vi "Swp_Main.vi"() -> ()   [LabVIEW 2024]
panel:
  out "输出日志 log":string
  in  "响应端口额外频率位移":i8(ring) items=["-2次基波"=-2, "-1次基波"=-1, "无位移"=0, "+1次基波"=1, "+2次基波"=2, "对称-2次基波"=98, "对称-1次基波"=99, "对称"=100, "对称+1次基波"=101, "对称+2次基波"=102]
  in  "响应(2号)端口类型":u8(ring) items=["单相", "三相αβ系", "三相同步系", "三相正负序"]
  in  "测量模式":u8(ring)=1 items=["仅测量信号", "扫频"]
  in  "与DSP连接的串口":refnum<visa-resource-name>
  in  "同步相位来源":u8(ring) items=["1号A相", "2号A相"]
  in  "检验示波器":bool
  in  "错误常量":errorcluster
  in  "DSP同时注入频点数":u32=5 min=1 max=20
  out "csv中存储列分别为":string
  in  "触发方向":u16(ring)=2 items=["Rising"=2, "Falling"=3]
  in  "触发阈值 (V)":dbl min=-20.0 max=20.0
  in  "示波器量程":u16(ring)=10 items=["20 mV"=1, "50 mV"=2, "100 mV"=3, "200 mV"=4, "500 mV"=5, "1 V"=6, "2 V"=7, "5 V"=8, "10 V"=9, "20 V"=10]
  out "测试选项说明":string
  in  "基波频率 f_fun":u32=50 min=1 max=100000
  in  "注入(1号)端口类型":u8(ring) items=["单相", "三相αβ系", "三相同步系", "三相正负序"]
  in  "实际幅值 Amp":u8(ring)=1 items=["= Amp0", "= Amp0 / freq"]
  in  "默认幅值 Amp0":u8(ring)=2 items=["10.0", "5.0", "1.0", "0.5", "0.1", "0.05", "0.01"]
  in  "等待稳态时间":dbl=0.04 min=1e-06 max=1.0
  out "Pha":cluster{dbl[], dbl[]}[](graph)
  out "Mag":cluster{dbl[], dbl[]}[](graph)
  in  "stop":bool
  out "PICOerror":bool
  in  "开始扫频":bool
  in  "总电源":bool=TRUE
  out "可以正常测量":bool
  out "正在扫频":bool
  in  "幅值显示方式":u8(ring) items=["dB", "abs"]
  in  "测量周期数 n":u32=2 min=1 max=10
  in  "同步频率上限 f_tick_ref":u32=1 min=1 max=50
  out "单频点最大使用内存":u64 caption="单频点最大使用内存(kS)"
  out "扫频点预览":cluster{"freqs":i32[], "freqs":dbl[]}[](graph)
  out "实际有效频点数 N":i32
  in  "密集中心频率 f_dens":u32=50 min=1 max=1000000
  in  "密度常数 dens":dbl min=0.0 max=50.0
  out "扫频点报告":string
  in  "期望频点数 N0":u32=20 min=2
  in  "频率下限 f_min":u32=10 min=1 max=500000
  in  "频率上限 f_max":u32=5000 min=10 max=1000000
  # "版本：v1.1 允许异性端口的扫频。允许在DSP或PICO未连接时跳过通信或采样环节。"
  # "如果你后续要增加端口类型选项，请不要改动现存项对应的取值。"
  # "操作面板"
  # "频点生成设置"
  # "频点采样设置"
  # "响应测试模式设置"
  # "示波器设置"
  # "基础设置\n实际频点生成也与测试模式相关。"
  # "Hz"
  # "程序总开关"
  # "频率越低，耗时越长。精度越高。"
  # "Hz"
  # "Hz"
  # "kS"
  # "完成设置后，按下以扫频。\n期间锁定操作。"
  # "Hz"
  # "默认测量所有4通道。\n\n例如，在测量 2500 Hz 响应时，\n总时长可以是 1 s，也可以是 1e-3 s。\n\nf_tick_ref 表示采样总时长的下限。\n不建议设置高于低频次谐波。"
  # "密度设置（测试功能）\n设为 dens<1.0 以禁用"
  # "通信设置"
  # "V"
  # "Hz"
  # "强制退出扫频。它不会被锁"
  # "s"
  # "杂项输出显示"
  # "扫频结果显示"
  # "测试面板，仅供开发过程中使用。"
  # "存储至csv时总是abs."
  # "与DSP间通信方式：\n\n开启串口\n送出1字节FFFF，以提醒DSP，接下来要进入允许输出的模式\n等待回应1字节（内容不限），以确认已建立联系\n\n第k次扫频循环中：\n送出1字节FF00，以提醒DSP，接下来要输出一组频率\n第1频点A相频率输出（1字节，16位无符号整型）\n第1频点A相幅值输出（2字节，32位浮点数）\n第1频点A相相位输出（1字节，16位无符号整型，360角度制）\n第1频点B相频率\n第1频点B相幅值\n第1频点B相相位\n第1频点C相频率\n第1频点C相幅值\n第1频点C相相位\n第2频点……\n……\n第n频点……\n送出1字节FF00，以表示这一组频点已经发送完毕\n等待DSP回应1字节，确认DSP已收到指令\n等待一段时间，该时间可在主界面内设置\n\n送出1字节F000，以提醒DSP，接下来要结束了\n等待DSP回应1字节，确认DSP知道要关闭了\n关闭串口\n\n备注：如果已知DSP可接收的最大频点数，请设置在该界面内。\n通信中，多余的频点位会用全0补齐。"
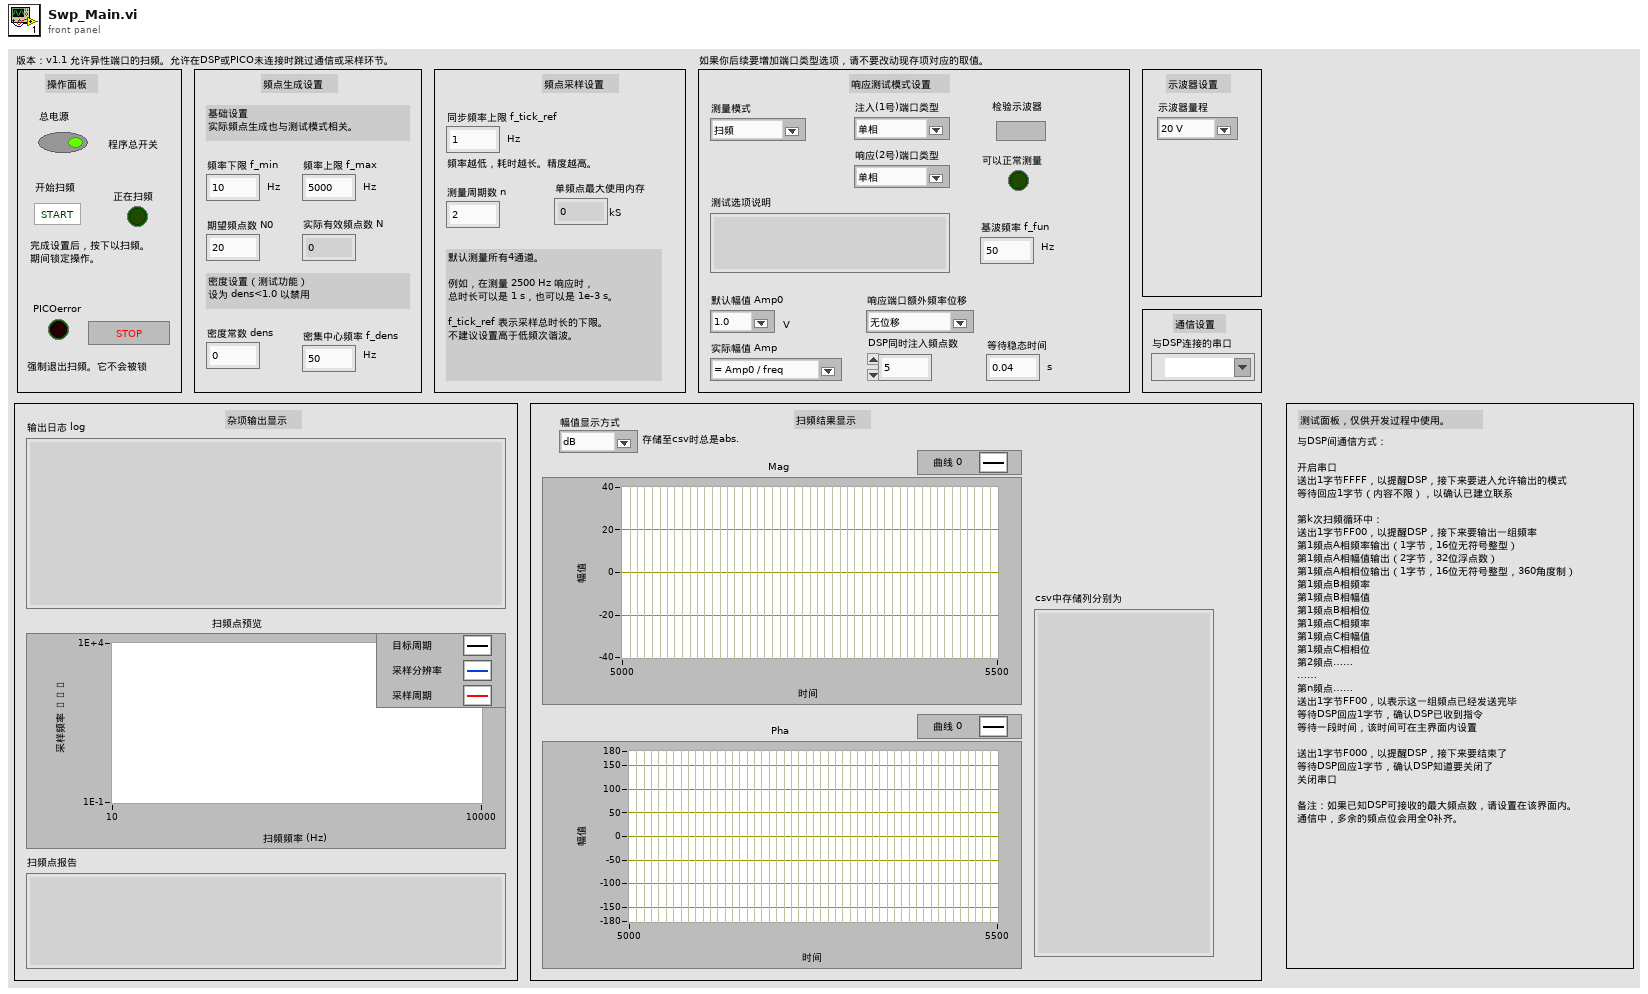
[diagram p1: front panel]
types:
  T1 = enum8{"Enabled", "Disabled", "Disabled and Grayed Out"}
  T2 = cluster{u32, u32, u32, dbl, u32, u8, u8, u8, u32, u32, u32, u32}
  T3 = enum16{"open", "replace", "create", "open or create", "replace or create", "replace or create with confirmation"}
  T4 = cluster{"Device Info":cluster{"Driver Version":string, "USB Version":string, "Hardware":string, "Variant":string, "Batch and Serial":string, "Cal Date":string, "Kernel Version":string, "Digital HW Version":string, "Analogue HW Version":string, "Firmware 1":string, "Firmware 2":string, "MSO":bool, "Number of Channels":i16}, "error out":errorcluster, "handle out":i16, "Enabled Array":i16[], "Max Adc value":i16}[]
  T5 = cluster{"Device Info":cluster{"Driver Version":string, "USB Version":string, "Hardware":string, "Variant":string, "Batch and Serial":string, "Cal Date":string, "Kernel Version":string, "Digital HW Version":string, "Analogue HW Version":string, "Firmware 1":string, "Firmware 2":string, "MSO":bool, "Number of Channels":i16}, "error out":errorcluster, "handle out":i16, "Enabled Array":i16[], "Max Adc value":i16}
  T6 = cluster{"Driver Version":string, "USB Version":string, "Hardware":string, "Variant":string, "Batch and Serial":string, "Cal Date":string, "Kernel Version":string, "Digital HW Version":string, "Analogue HW Version":string, "Firmware 1":string, "Firmware 2":string, "MSO":bool, "Number of Channels":i16}
  T7 = cluster{"Device Info":cluster{"Driver Version":string, "USB Version":string, "Hardware":string, "Variant":string, "Batch and Serial":string, "Cal Date":string, "Kernel Version":string, "Digital HW Version":string, "Analogue HW Version":string, "Firmware 1":string, "Firmware 2":string, "MSO":bool, "Number of Channels":i16}, "Enabled Array":i16[], "handle out":i16, "error out":errorcluster}
  T8 = cluster{"Channel A Buffer":i16[], "Channel B Buffer":i16[], "Channel C Buffer":i16[], "Channel D Buffer":i16[], "Channel E Buffer":i16[], "Channel F Buffer":i16[], "Channel G Buffer":i16[], "Channel H Buffer":i16[], "Port 0 Buffer":i16[], "Port 1 Buffer":i16[]}[]
  T9 = typedef "PicoBuffers.ctl" = cluster{"Max Buffer Pointers":u64[][][], "Min Buffer Pointers":u64[][][], "StreamingDataInfo":cluster{"Channel":u32, "Down-Sample Mode":u32, "PICO_DATA_TYPE":enum32{"PICO_INT8_T", "PICO_INT16_T", "PICO_INT32_T", "PICO_UINT32_T", "PICO_INT64_T", ""}, "Samples":i32, "bufferIndex":u64, "startIndex":i32, "overflow":i16}[][]}
  T10 = cluster{"Data Pointers":T9, "error out":errorcluster, "handle out":i16}
  T11 = cluster{"Data":dbl[], "Data":dbl[], "Data":dbl[], "Data":dbl[], "Data":dbl[], "Data":dbl[]}
  T12 = cluster{"Data Pointers":T9, "Enabled Array":i16[], "error out":errorcluster, "handle out":i16}
  T13 = cluster{"Data Pointers":T9, "Enabled Array":i16[], "error out":errorcluster, "handle out":i16}[]
  T14 = cluster{"Value":u32, "Value":u32, "Value":u32, "Value":dbl, "Value":u32, "Value":u8, "Value":u8, "Value":u8, "Value":u32, "Value":u32, "Value":u32, "Value":u32}
  T15 = cluster{bool, bool, bool, bool, bool, bool, bool, bool, bool, bool, bool, bool}
  T16 = cluster{"freqs, measu, measu comp":i32[], dbl[]}[]
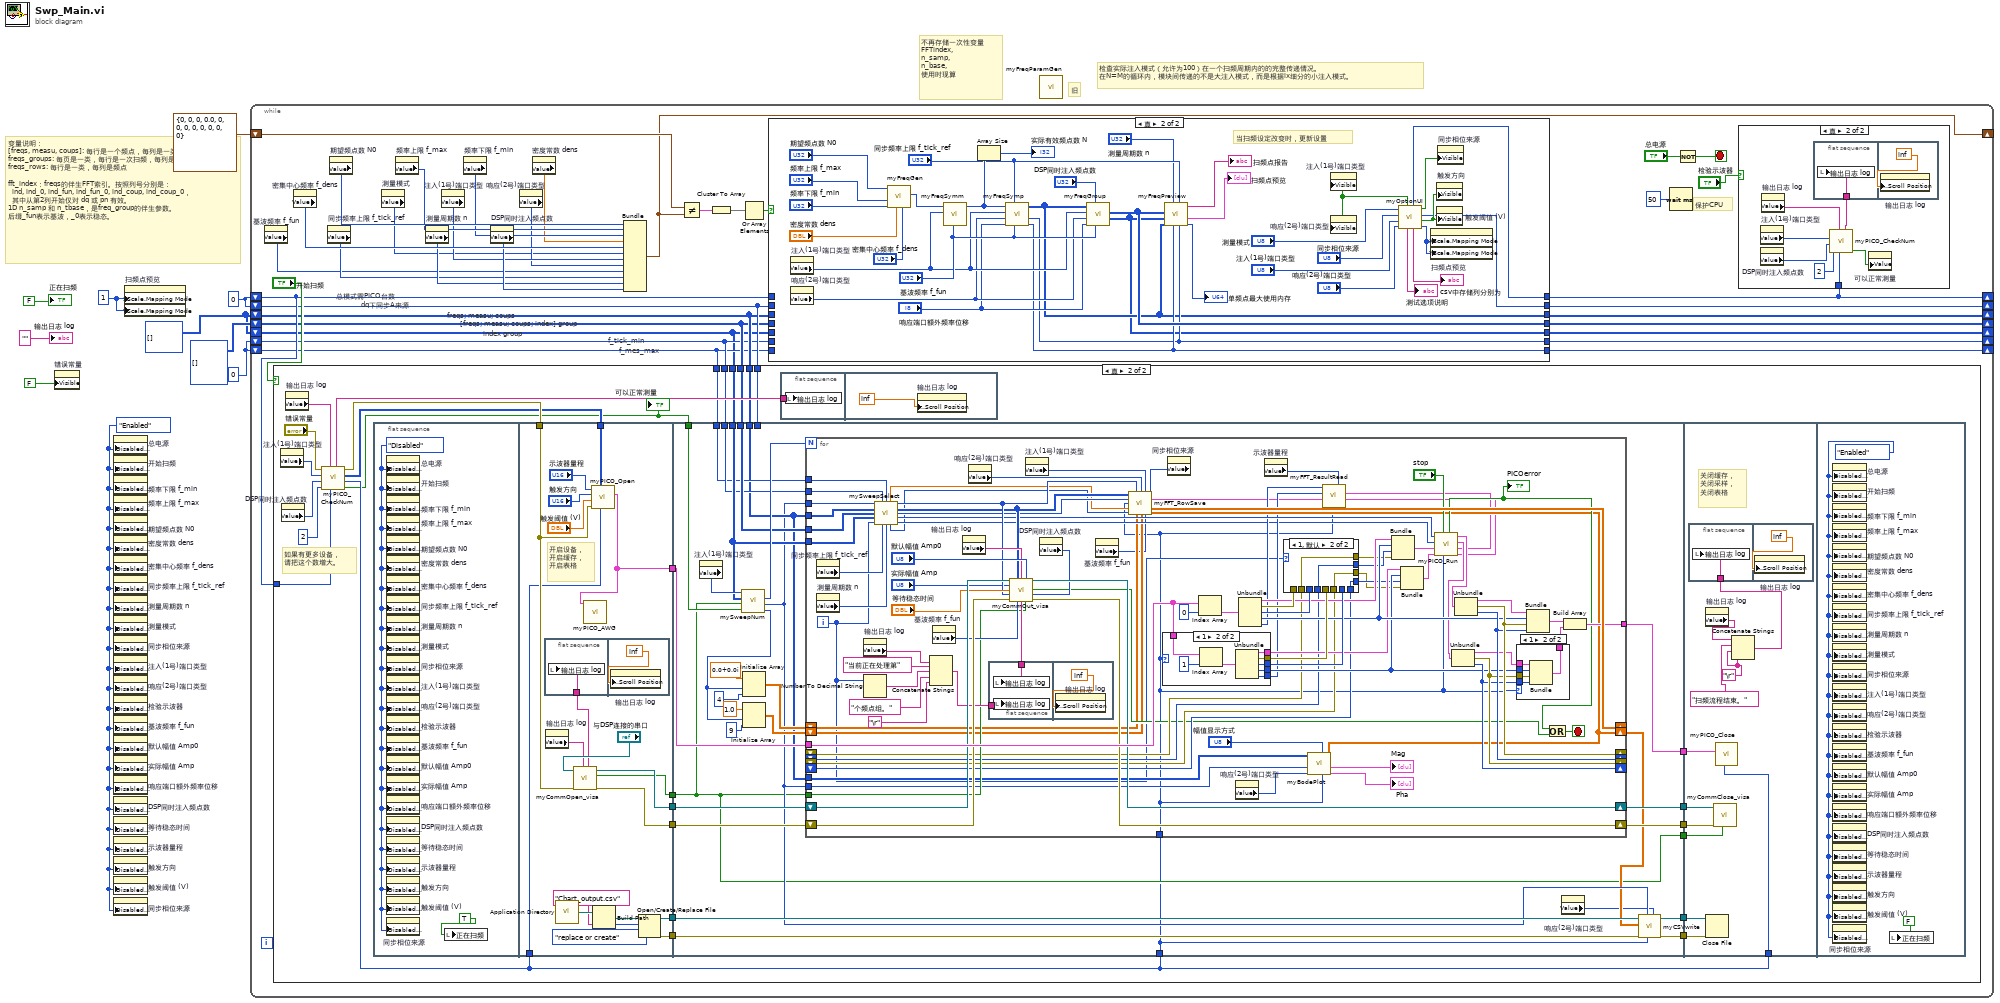
[diagram p0: block diagram]
diagram:
  w3 = u32 0
  w5 = u8 1 ("X标尺.映射模式")
  w6 = T1."Enabled" ("禁用")
  w8 = u8 0
  w1 = i32[][] []
  # "不再存储一次性变量\nFFTindex, \nn_samp, \nn_base, \n使用时现算"
  # "检查实际注入模式（允许为100）在一个扫频周期内的的完整传递情况。\n在N=M的循环内，模块间传递的不是大注入模式，而是根据ix细分的小注入模式。"
  # "旧"
  # "变量说明：\n[freqs, measu, coups]: 每行是一个频点，每列是一类\nfreqs_groups: 每页是一类，每行是一次扫频，每列是频点\nfreqs_rows: 每行是一类，每列是频点\n\nfft_index：freqs的伴生FFT索引。按照列号分别是：\n  ind, ind_0, ind_fun, ind_fun_0, ind_coup, ind_coup_0，\n  其中从第2列开始仅对 dq 或 pn 有效。\n1D n_samp 和 n_tbase，是freq_group的伴生参数。\n后缀_fun表示基波，_0表示稳态。"
  n1 = property on="错误常量" class="Clust (严格)"("Visible"=FALSE ("可见")) -> ()  [unwired: 2 in, 2 out]
  n2 = property on="总电源" class="Bool"("DisabledEnum"=w6) -> ()  [unwired: 2 in, 2 out]
  n3 = property on="开始扫频" class="Bool"("DisabledEnum"=w6) -> ()  [unwired: 2 in, 2 out]
  n4 = property on="频率下限 f_min" class="DigNum (严格)"("DisabledEnum"=w6) -> ()  [unwired: 2 in, 2 out]
  n5 = property on="频率上限 f_max" class="DigNum (严格)"("DisabledEnum"=w6) -> ()  [unwired: 2 in, 2 out]
  n6 = property on="期望频点数 N0" class="DigNum (严格)"("DisabledEnum"=w6) -> ()  [unwired: 2 in, 2 out]
  n7 = property on="密度常数 dens" class="DigNum (严格)"("DisabledEnum"=w6) -> ()  [unwired: 2 in, 2 out]
  n8 = property on="密集中心频率 f_dens" class="DigNum (严格)"("DisabledEnum"=w6) -> ()  [unwired: 2 in, 2 out]
  n9 = property on="同步频率上限 f_tick_ref" class="DigNum (严格)"("DisabledEnum"=w6) -> ()  [unwired: 2 in, 2 out]
  n10 = property on="测量周期数 n" class="DigNum (严格)"("DisabledEnum"=w6) -> ()  [unwired: 2 in, 2 out]
  n11 = property on="测量模式" class="Ring (严格)"("DisabledEnum"=w6) -> ()  [unwired: 2 in, 2 out]
  n12 = property on="同步相位来源" class="Ring (严格)"("DisabledEnum"=w6) -> ()  [unwired: 2 in, 2 out]
  n13 = property on="注入(1号)端口类型" class="Ring (严格)"("DisabledEnum"=w6) -> ()  [unwired: 2 in, 2 out]
  n14 = property on="响应(2号)端口类型" class="Ring (严格)"("DisabledEnum"=w6) -> ()  [unwired: 2 in, 2 out]
  n15 = property on="检验示波器" class="Bool"("DisabledEnum"=w6) -> ()  [unwired: 2 in, 2 out]
  n16 = property on="基波频率 f_fun" class="DigNum (严格)"("DisabledEnum"=w6) -> ()  [unwired: 2 in, 2 out]
  n17 = property on="默认幅值 Amp0" class="Ring (严格)"("DisabledEnum"=w6) -> ()  [unwired: 2 in, 2 out]
  n18 = property on="实际幅值 Amp" class="Ring (严格)"("DisabledEnum"=w6) -> ()  [unwired: 2 in, 2 out]
  n19 = property on="响应端口额外频率位移" class="Ring (严格)"("DisabledEnum"=w6) -> ()  [unwired: 2 in, 2 out]
  n20 = property on="DSP同时注入频点数" class="DigNum (严格)"("DisabledEnum"=w6) -> ()  [unwired: 2 in, 2 out]
  n21 = property on="等待稳态时间" class="DigNum (严格)"("DisabledEnum"=w6) -> ()  [unwired: 2 in, 2 out]
  n22 = property on="示波器量程" class="Ring (严格)"("DisabledEnum"=w6) -> ()  [unwired: 2 in, 2 out]
  n23 = property on="触发方向" class="Ring (严格)"("DisabledEnum"=w6) -> ()  [unwired: 2 in, 2 out]
  n24 = property on="触发阈值 (V)" class="DigNum (严格)"("DisabledEnum"=w6) -> ()  [unwired: 2 in, 2 out]
  n25 = property on="同步相位来源" class="Ring (严格)"("DisabledEnum"=w6) -> ()  [unwired: 2 in, 2 out]
  n26 = property on="扫频点预览" class="XYGraph (严格)"("XScale.Mapping Mode"=w5, "YScale.Mapping Mode"=w5) -> ()  [unwired: 2 in, 2 out]
  n27 = while {
    shift-right: [w37] -> _
    shift-left: T2 {0, 0, 0, 0.0, 0, 0, 0, 0, 0, 0, 0, 0} -> [w38]
    shift-right: [w32] -> _
    shift-left: w1 -> [w17]
    shift-right: [w24] -> _
    shift-left: w8 -> [w20]
    shift-right: [w23] -> _
    shift-left: w8 -> [w18]
    shift-right: [w22] -> _
    shift-left: w3 -> [w15]
    shift-right: [w21] -> _
    shift-left: w3 -> [w14]
    shift-right: [w19] -> _
    shift-left: i32[][][] [] -> [w16]
    shift-right: [w13] -> _
    shift-left: w1 -> [w12]
    stop <- w45 stop-if-true
    # "index group"
    # "f_mes_max"
    # "f_tick_min"
    # "[freqs; measu; coups; index] group"
    # "freqs; measu; coups"
    # "总模式需PICO台数"
    # "dq下同步A来源"
    # "保护CPU"
    n28 = property on="基波频率 f_fun" class="DigNum (严格)"() -> ("Value"=w28:u32)  [unwired: 2 in, 2 out]
    n29 = case shown="真" "开始扫频" {
      tunnel: w20 -> [_ w118]
      tunnel: w18 -> [_ w98]
      tunnel: w17 -> [_ w99]
      tunnel: w16 -> [_ w100]
      tunnel: w15 -> [_ w101]
      tunnel: w14 -> [_ w102]
      tunnel: w12 -> [_ w103]
      frame False {
      }
      frame True {
        # "如果有更多设备，\n请把这个数增大。"
        n30 = property on="注入(1号)端口类型" class="Ring (严格)"() -> ("Value"=w122:u8)  [unwired: 2 in, 2 out]
        n31 = property on="DSP同时注入频点数" class="DigNum (严格)"() -> ("Value"=w121:u32)  [unwired: 2 in, 2 out]
        n32 = property on="输出日志 log" class="Str"() -> ("Value"=w120:string)  [unwired: 2 in, 2 out]
        n33 = call "myPICO_CheckNum.vi"("需要的示波器台数"=w118, "当前log"=w120, "最大检测设备数"=i16 2, "最大同时扫频数"=w121, "注入(1号)端口类型"=w122, "错误常量"="错误常量") -> ("可以正常测量"=w104:bool, "实际驱动设备数"=w105:u16, "序列号组 2"=w123:i8[][], "错误输出"=w124:errorcluster, "更新log"=w119:string)  [unwired: 1 in]
        "可以正常测量" <- w104
        n34 = flat-sequence {
          tunnel: w123 -> [w147]
          tunnel: w124 -> [w137]
          tunnel: [w133] -> w117
          tunnel: [w139] -> w116
          tunnel: [w138] -> w115
          tunnel: [w135] -> w114
          tunnel: [w134] -> w113
          tunnel: w105 -> [w130]
          tunnel: [w129] -> w112
          tunnel: w117 -> [w174]
          tunnel: w105 -> [w150]
          tunnel: [w173] -> w111
          tunnel: w116 -> [w165]
          tunnel: w115 -> [w172]
          tunnel: [w166] -> w110
          tunnel: [w171] -> w109
          tunnel: w114 -> [w170]
          tunnel: w113 -> [w169]
          tunnel: [w168] -> w108
          tunnel: [w167] -> w107
          tunnel: w112 -> [w152]
          tunnel: [w152] -> w106
          tunnel: w104 -> [w162]
          tunnel: w103 -> [w160]
          tunnel: w102 -> [w158]
          tunnel: w101 -> [w159]
          tunnel: w100 -> [w161]
          tunnel: w99 -> [w157]
          tunnel: w98 -> [_]
          tunnel: w105 -> [w295]
          tunnel: w111 -> [w305]
          tunnel: w110 -> [w304]
          tunnel: w109 -> [w303]
          tunnel: w108 -> [w302]
          tunnel: w107 -> [w301]
          tunnel: w106 -> [w296]
          frame #0 {
            w128 = T1."Disabled" ("禁用")
            n35 = property on="总电源" class="Bool"("DisabledEnum"=w128) -> ()  [unwired: 2 in, 2 out]
            n36 = property on="开始扫频" class="Bool"("DisabledEnum"=w128) -> ()  [unwired: 2 in, 2 out]
            n37 = property on="频率下限 f_min" class="DigNum (严格)"("DisabledEnum"=w128) -> ()  [unwired: 2 in, 2 out]
            n38 = property on="频率上限 f_max" class="DigNum (严格)"("DisabledEnum"=w128) -> ()  [unwired: 2 in, 2 out]
            n39 = property on="期望频点数 N0" class="DigNum (严格)"("DisabledEnum"=w128) -> ()  [unwired: 2 in, 2 out]
            n40 = property on="密度常数 dens" class="DigNum (严格)"("DisabledEnum"=w128) -> ()  [unwired: 2 in, 2 out]
            n41 = property on="密集中心频率 f_dens" class="DigNum (严格)"("DisabledEnum"=w128) -> ()  [unwired: 2 in, 2 out]
            n42 = property on="同步频率上限 f_tick_ref" class="DigNum (严格)"("DisabledEnum"=w128) -> ()  [unwired: 2 in, 2 out]
            n43 = property on="测量周期数 n" class="DigNum (严格)"("DisabledEnum"=w128) -> ()  [unwired: 2 in, 2 out]
            n44 = property on="测量模式" class="Ring (严格)"("DisabledEnum"=w128) -> ()  [unwired: 2 in, 2 out]
            n45 = property on="同步相位来源" class="Ring (严格)"("DisabledEnum"=w128) -> ()  [unwired: 2 in, 2 out]
            n46 = property on="注入(1号)端口类型" class="Ring (严格)"("DisabledEnum"=w128) -> ()  [unwired: 2 in, 2 out]
            n47 = property on="响应(2号)端口类型" class="Ring (严格)"("DisabledEnum"=w128) -> ()  [unwired: 2 in, 2 out]
            n48 = property on="检验示波器" class="Bool"("DisabledEnum"=w128) -> ()  [unwired: 2 in, 2 out]
            n49 = property on="基波频率 f_fun" class="DigNum (严格)"("DisabledEnum"=w128) -> ()  [unwired: 2 in, 2 out]
            n50 = property on="默认幅值 Amp0" class="Ring (严格)"("DisabledEnum"=w128) -> ()  [unwired: 2 in, 2 out]
            n51 = property on="实际幅值 Amp" class="Ring (严格)"("DisabledEnum"=w128) -> ()  [unwired: 2 in, 2 out]
            n52 = property on="响应端口额外频率位移" class="Ring (严格)"("DisabledEnum"=w128) -> ()  [unwired: 2 in, 2 out]
            n53 = property on="DSP同时注入频点数" class="DigNum (严格)"("DisabledEnum"=w128) -> ()  [unwired: 2 in, 2 out]
            n54 = property on="等待稳态时间" class="DigNum (严格)"("DisabledEnum"=w128) -> ()  [unwired: 2 in, 2 out]
            n55 = property on="示波器量程" class="Ring (严格)"("DisabledEnum"=w128) -> ()  [unwired: 2 in, 2 out]
            n56 = property on="触发方向" class="Ring (严格)"("DisabledEnum"=w128) -> ()  [unwired: 2 in, 2 out]
            n57 = property on="触发阈值 (V)" class="DigNum (严格)"("DisabledEnum"=w128) -> ()  [unwired: 2 in, 2 out]
            n58 = property on="同步相位来源" class="Ring (严格)"("DisabledEnum"=w128) -> ()  [unwired: 2 in, 2 out]
            n59 = local write "正在扫频"(TRUE) -> ()
          }
          frame #1 {
            # "开启设备，\n开启缓存，\n开启表格"
            n60 = flat-sequence {
              tunnel: w131 -> [w148]
              frame #0 {
                n61 = local write "输出日志 log"(w148) -> ()
              }
              frame #1 {
                n62 = property on="输出日志 log" class="Str"("Text.Scroll Position"=inf) -> ()  [unwired: 2 in, 2 out]
              }
            }
            n63 = property on="输出日志 log" class="Str"() -> ("Value"=w132:string)  [unwired: 2 in, 2 out]
            n64 = call <vilib>:"Application Directory.vi"() -> ("Application Directory"=w142:path)
            n65 = call "myCommOpen_visa.vi"("log输入"=w132, "错误输入（无错误）"=w137, "与DSP连接的串口"="与DSP连接的串口") -> ("错误输出"=w134:errorcluster, "是否有可用DSP"=w129:bool, "VISA resource name out"=w135:refnum<visa-resource-name>, "log输出"=w131:string)  [unwired: 5 in]
            n66 = call "myPICO_Open.vi"("需要台数"=w130, "serials"=w147, "错误输入（无错误）"=w137, "触发阈值 (V)"="触发阈值 (V)", "触发方向"="触发方向", "示波器量程"="示波器量程") -> ("数组"=w133:T4)  [unwired: 5 in]
            n67 = call "myPICO_AWG.vi"("数组"=w133) -> ()  [unwired: 11 in]
            n68 = Build Path(base path=w142, name or relative path="Chart_output.csv" ("name (excel)")) -> (appended path=w141:path)
            n69 = Open/Create/Replace File(file path (use dialog)=w141, operation (0:open)=T3."replace or create" ("操作(0:open)")) -> (refnum out=w139:refnum<file>, error out=w138:errorcluster)  [unwired: 4 in, 1 out]
          }
          frame #2 {
            n70 = property on="注入(1号)端口类型" class="Ring (严格)"() -> ("Value"=w163:u8)  [unwired: 2 in, 2 out]
            n71 = call "mySweepNum.vi"("可以正常测量"=w162, "是否有可用DSP"=w152, "index group"=w160, "注入(1号)端口类型"=w163) -> ("频点数"=w156:i32, "实际使用的注入模式"=w154:u8, "M"=w164:i32)  [unwired: 5 in]
            n72 = Initialize Array(cdb 0.0+0.0i, w156, 4 ("维数大小")) -> (w176:cdb[][])
            n73 = Initialize Array(1.0 ("元素"), w156, 9 ("维数大小")) -> (w175:dbl[][])
            n74 = for {
              N: w164 -> [_]
              shift-right: [w270] -> _
              shift-left: w176 -> [w186]
              shift-right: [w202] -> w153
              shift-left: w175 -> [w187]
              shift-right: [w269] -> _
              shift-left: _ -> [w207]
              shift-right: [w268] -> _
              shift-left: _ -> [w206]
              shift-right: [w267] -> _
              shift-left: _ -> [w205]
              shift-right: [w266] -> _
              shift-left: _ -> [w204]
              tunnel: w150 -> [w180]
              tunnel: w174 -> [w264]
              tunnel: [w265] -> w173
              shift-right: [w256] -> w167
              shift-left: w170 -> [w261]
              shift-right: [w257] -> w168
              shift-left: w169 -> [w260]
              tunnel: w152 -> [w213]
              tunnel: w154 -> [w221]
              tunnel: w157 -> [w220]
              tunnel: w161 -> [w219]
              tunnel: w160 -> [w218]
              tunnel: w159 -> [w215]
              tunnel: w158 -> [w214]
              tunnel: w154 -> [w199]
              tunnel: w157 -> [w201]
              i -> [w181]
              stop <- w258 stop-if-true
              n75 = property on="同步频率上限 f_tick_ref" class="DigNum (严格)"() -> ("Value"=w217:u32)  [unwired: 2 in, 2 out]
              n76 = property on="测量周期数 n" class="DigNum (严格)"() -> ("Value"=w216:u32)  [unwired: 2 in, 2 out]
              n77 = property on="输出日志 log" class="Str"() -> ("Value"=w247:string)  [unwired: 2 in, 2 out]
              n78 = Number To Decimal String(number=w181) -> (decimal integer string=w255:string)  [unwired: 1 in]
              n79 = call "mySweepSelect.vi"("实际使用的注入模式"=w221, "f_tick_min"=w215, "f_mes_max"=w214, "freqs, measu. coups"=w220, "freqs groups"=w219, "index group"=w218, "ix"=w181, "同步频率上限 f_tick_ref"=w217, "测量周期数 n"=w216) -> ("f_tick"=w185:dbl, "注入小模式"=w212:u8, "freq rows"=w211:i32[][], "index row"=w210:i32[], "sample"=w208:u64, "f_mes"=w184:i32, "timebase"=w189:u32)
              n80 = Concatenate Strings(w247, "当前正在处理第", w255, "个频点组。", "\r") -> (w246:string)
              n81 = property on="基波频率 f_fun" class="DigNum (严格)"() -> ("Value"=w249:u32)  [unwired: 2 in, 2 out]
              n82 = property on="输出日志 log" class="Str"() -> ("Value"=w244:string)  [unwired: 2 in, 2 out]
              n83 = property on="响应(2号)端口类型" class="Ring (严格)"() -> ("Value"=w190:u8)  [unwired: 2 in, 2 out]
              n84 = flat-sequence {
                tunnel: w246 -> [w293]
                tunnel: w245 -> [w292]
                frame #0 {
                  n85 = local write "输出日志 log"(w292) -> ()
                  n86 = local write "输出日志 log"(w293) -> ()
                }
                frame #1 {
                  n87 = property on="输出日志 log" class="Str"("Text.Scroll Position"=inf) -> ()  [unwired: 2 in, 2 out]
                }
              }
              n88 = property on="注入(1号)端口类型" class="Ring (严格)"() -> ("Value"=w183:u8)  [unwired: 2 in, 2 out]
              n89 = property on="DSP同时注入频点数" class="DigNum (严格)"() -> ("Value"=w248:u32)  [unwired: 2 in, 2 out]
              n90 = call "myCommOut_visa.vi"("VISA资源名称"=w261, "freqs rows"=w211, "log输入"=w244, "默认幅值 Amp0"="默认幅值 Amp0", "实际幅值 Amp"="实际幅值 Amp", "t_wait"="等待稳态时间", "扰动注入模式"=w212, "最大同时扫频数"=w248, "错误输入（无错误）"=w260, "基波频率"=w249, "存在DSP"=w213) -> ("VISA资源名称 2"=w256:refnum<visa-resource-name>, "error out"=w203:bool, "log输出"=w245:string, "错误输出"=w257:errorcluster)  [unwired: 1 in]
              n91 = property on="基波频率 f_fun" class="DigNum (严格)"() -> ("Value"=w182:u32)  [unwired: 2 in, 2 out]
              n92 = case shown="1" w180 {
                tunnel: w264 -> [_ w291]
                tunnel: [_ w290] -> w231
                tunnel: [_ w289] -> w238
                tunnel: [_ w288] -> w236
                tunnel: [_ w287] -> w192
                tunnel: [_ w284] -> w230
                frame 0, Default {
                }
                frame 1 {
                  n93 = Index Array(array=w291, index=1 ("索引")) -> (element=w285:T5)
                  n94 = Unbundle(w285) -> ("Device Info"=w290:T6, "error out"=w289:errorcluster, "handle out"=w288:i16, "Enabled Array"=w284:i16[], "Max Adc value"=w287:i16)
                }
              }
              n95 = property on="同步相位来源" class="Ring (严格)"() -> ("Value"=w209:u8)  [unwired: 2 in, 2 out]
              n96 = Index Array(array=w264, index=0 ("索引")) -> (element=w242:T5)
              n97 = property on="响应(2号)端口类型" class="Ring (严格)"() -> ("Value"=w198:u8)  [unwired: 2 in, 2 out]
              n98 = Unbundle(w242) -> ("Device Info"=w235:T6, "error out"=w239:errorcluster, "handle out"=w237:i16, "Enabled Array"=w234:i16[], "Max Adc value"=w193:i16)
              n99 = property on="示波器量程" class="Ring (严格)"() -> ("Value"=w191:u16)  [unwired: 2 in, 2 out]
              n100 = case shown="1, 默认" w181 {
                tunnel: w239 -> [w274 _]
                tunnel: w207 -> [_ w278]
                tunnel: w237 -> [w273 _]
                tunnel: w206 -> [_ w277]
                tunnel: w238 -> [w272 _]
                tunnel: w205 -> [_ w276]
                tunnel: w236 -> [w271 _]
                tunnel: w204 -> [_ w275]
                tunnel: [w274 w278] -> w232
                tunnel: [w273 w277] -> w233
                tunnel: [w272 w276] -> w228
                tunnel: [w271 w275] -> w229
                frame 0 {
                }
                frame 1, Default {
                }
              }
              n101 = Bundle("Device Info"=w235, "Enabled Array"=w234, "handle out"=w233, "error out"=w232) -> (w227:T7)  [unwired: 1 in]
              n102 = Bundle("Device Info"=w231, "Enabled Array"=w230, "handle out"=w229, "error out"=w228) -> (w226:T7)  [unwired: 1 in]
              n103 = call "myPICO_Run.vi"("实际驱动台数"=w180, "stop"="stop", "簇 3"=w226, "簇 4"=w227, "n_tbase"=w189, "n_samp"=w208) -> ("MultiBuffers (Max or non-aggregated) 2"=w194:T8, "MultiBuffers (Max or non-aggregated)"=w195:T8, "簇 2"=w197:T10, "簇"=w225:T10, "布尔输出"=w259:bool)  [unwired: 1 in]
              "PICOerror" <- w259
              n104 = call "myFFT_ResultRead.vi"("MultiBuffers 2"=w194, "MultiBuffers 1"=w195, "示波器量程"=w191, "可用示波器数"=w180, "Max Adc value 2"=w192, "Max Adc value"=w193) -> ("输出簇"=w188:T11)  [unwired: 5 in]
              n105 = call "myFFT_RowSave.vi"("freqs rows"=w211, "小注入模式"=w212, "响应模式"=w190, "注入(1号)端口类型"=w183, "dq同步来源"=w209, "index row"=w210, "采样结果簇"=w188, "可用pico数(仅用于模式100)"=w180, "f_tick"=w185, "f_mes"=w184, "稳态工作点输入"=w186, "写表结果输入"=w187, "基波频率 f_fun"=w182) -> ("稳态工作点输出"=w270:cdb[][], "写表结果输出"=w202:dbl[][])  [unwired: 1 in]
              n106 = call "myBodePlot.vi"("swp_data"=w202, "可用pico数"=w180, "幅值单位"="幅值显示方式", "响应选项"=w198, "注入选项"=w199, "freqs, meas, coups"=w201) -> ("Pha"=→"Pha":cluster{dbl[], dbl[]}[], "Mag"=→"Mag":cluster{dbl[], dbl[]}[])  [unwired: 4 in]
              n107 = Unbundle(w197) -> ("Data Pointers"=w224:T9, "error out"=w267:errorcluster, "handle out"=w266:i16)
              n108 = Unbundle(w225) -> ("Data Pointers"=w223:T9, "error out"=w269:errorcluster, "handle out"=w268:i16)
              n109 = case shown="1" w180 {
                tunnel: [_ w283] -> w241
                tunnel: w224 -> [_ w282]
                tunnel: w230 -> [_ w281]
                tunnel: w267 -> [_ w280]
                tunnel: w266 -> [_ w279]
                frame 0, Default {
                }
                frame 1 {
                  n110 = Bundle("Data Pointers"=w282, "Enabled Array"=w281, "error out"=w280, "handle out"=w279) -> (w283:T12)  [unwired: 1 in]
                }
              }
              n111 = Bundle("Data Pointers"=w223, "Enabled Array"=w234, "error out"=w269, "handle out"=w268) -> (w240:T12)  [unwired: 1 in]
              n112 = Or(x=w259, y=w203) -> (x .or. y?=w258:bool)
              n113 = Build Array(w240, w241) -> (w265:T13)
            }
            n114 = property on="响应(2号)端口类型" class="Ring (严格)"() -> ("Value"=w151:u8)  [unwired: 2 in, 2 out]
            n115 = call "myCSVwrite.vi"("响应选项"=w151, "可用PICO数"=w150, "注入选项"=w154, "错误输入（无错误）"=w172, "写表结果输入"=w153, "字节流文件输入"=w165) -> ("错误输出"=w171:errorcluster, "字节流文件输出"=w166:refnum<file>)  [unwired: 4 in]
          }
          frame #3 {
            w299 = "\r"
            # "关闭缓存，\n关闭采样，\n关闭表格"
            n116 = flat-sequence {
              tunnel: w297 -> [w306]
              frame #0 {
                n117 = local write "输出日志 log"(w306) -> ()
              }
              frame #1 {
                n118 = property on="输出日志 log" class="Str"("Text.Scroll Position"=inf) -> ()  [unwired: 2 in, 2 out]
              }
            }
            n119 = property on="输出日志 log" class="Str"() -> ("Value"=w298:string)  [unwired: 2 in, 2 out]
            n120 = Close File(refnum=w304, error in=w303) -> ()  [unwired: 2 out]
            n121 = call "myCommClose_visa.vi"("是否存在DSP"=w296, "错误输入（无错误）"=w302, "VISA资源名称"=w301) -> ()  [unwired: 8 in, 1 out]
            n122 = call "myPICO_Close.vi"("数值"=w295, "数组"=w305) -> ()  [unwired: 10 in]
            n123 = Concatenate Strings(w298, "扫频流程结束。", w299, w299) -> (w297:string)
          }
          frame #4 {
            w309 = T1."Enabled" ("禁用")
            n124 = property on="总电源" class="Bool"("DisabledEnum"=w309) -> ()  [unwired: 2 in, 2 out]
            n125 = property on="开始扫频" class="Bool"("DisabledEnum"=w309) -> ()  [unwired: 2 in, 2 out]
            n126 = property on="频率下限 f_min" class="DigNum (严格)"("DisabledEnum"=w309) -> ()  [unwired: 2 in, 2 out]
            n127 = property on="频率上限 f_max" class="DigNum (严格)"("DisabledEnum"=w309) -> ()  [unwired: 2 in, 2 out]
            n128 = property on="期望频点数 N0" class="DigNum (严格)"("DisabledEnum"=w309) -> ()  [unwired: 2 in, 2 out]
            n129 = property on="密度常数 dens" class="DigNum (严格)"("DisabledEnum"=w309) -> ()  [unwired: 2 in, 2 out]
            n130 = property on="密集中心频率 f_dens" class="DigNum (严格)"("DisabledEnum"=w309) -> ()  [unwired: 2 in, 2 out]
            n131 = property on="同步频率上限 f_tick_ref" class="DigNum (严格)"("DisabledEnum"=w309) -> ()  [unwired: 2 in, 2 out]
            n132 = property on="测量周期数 n" class="DigNum (严格)"("DisabledEnum"=w309) -> ()  [unwired: 2 in, 2 out]
            n133 = property on="测量模式" class="Ring (严格)"("DisabledEnum"=w309) -> ()  [unwired: 2 in, 2 out]
            n134 = property on="同步相位来源" class="Ring (严格)"("DisabledEnum"=w309) -> ()  [unwired: 2 in, 2 out]
            n135 = property on="注入(1号)端口类型" class="Ring (严格)"("DisabledEnum"=w309) -> ()  [unwired: 2 in, 2 out]
            n136 = property on="响应(2号)端口类型" class="Ring (严格)"("DisabledEnum"=w309) -> ()  [unwired: 2 in, 2 out]
            n137 = property on="检验示波器" class="Bool"("DisabledEnum"=w309) -> ()  [unwired: 2 in, 2 out]
            n138 = property on="基波频率 f_fun" class="DigNum (严格)"("DisabledEnum"=w309) -> ()  [unwired: 2 in, 2 out]
            n139 = property on="默认幅值 Amp0" class="Ring (严格)"("DisabledEnum"=w309) -> ()  [unwired: 2 in, 2 out]
            n140 = property on="实际幅值 Amp" class="Ring (严格)"("DisabledEnum"=w309) -> ()  [unwired: 2 in, 2 out]
            n141 = property on="响应端口额外频率位移" class="Ring (严格)"("DisabledEnum"=w309) -> ()  [unwired: 2 in, 2 out]
            n142 = property on="DSP同时注入频点数" class="DigNum (严格)"("DisabledEnum"=w309) -> ()  [unwired: 2 in, 2 out]
            n143 = property on="等待稳态时间" class="DigNum (严格)"("DisabledEnum"=w309) -> ()  [unwired: 2 in, 2 out]
            n144 = property on="示波器量程" class="Ring (严格)"("DisabledEnum"=w309) -> ()  [unwired: 2 in, 2 out]
            n145 = property on="触发方向" class="Ring (严格)"("DisabledEnum"=w309) -> ()  [unwired: 2 in, 2 out]
            n146 = property on="触发阈值 (V)" class="DigNum (严格)"("DisabledEnum"=w309) -> ()  [unwired: 2 in, 2 out]
            n147 = property on="同步相位来源" class="Ring (严格)"("DisabledEnum"=w309) -> ()  [unwired: 2 in, 2 out]
            n148 = local write "正在扫频"(FALSE) -> ()
          }
        }
        n149 = flat-sequence {
          tunnel: w119 -> [w310]
          frame #0 {
            n150 = local write "输出日志 log"(w310) -> ()
          }
          frame #1 {
            n151 = property on="输出日志 log" class="Str"("Text.Scroll Position"=inf) -> ()  [unwired: 2 in, 2 out]
          }
        }
      }
    }
    n152 = property on="密集中心频率 f_dens" class="DigNum (严格)"() -> ("Value"=w39:u32)  [unwired: 2 in, 2 out]
    n153 = property on="同步频率上限 f_tick_ref" class="DigNum (严格)"() -> ("Value"=w29:u32)  [unwired: 2 in, 2 out]
    n154 = property on="期望频点数 N0" class="DigNum (严格)"() -> ("Value"=w43:u32)  [unwired: 2 in, 2 out]
    n155 = property on="测量模式" class="Ring (严格)"() -> ("Value"=w25:u8)  [unwired: 2 in, 2 out]
    n156 = property on="频率上限 f_max" class="DigNum (严格)"() -> ("Value"=w42:u32)  [unwired: 2 in, 2 out]
    n157 = property on="测量周期数 n" class="DigNum (严格)"() -> ("Value"=w30:u32)  [unwired: 2 in, 2 out]
    n158 = property on="注入(1号)端口类型" class="Ring (严格)"() -> ("Value"=w27:u8)  [unwired: 2 in, 2 out]
    n159 = property on="频率下限 f_min" class="DigNum (严格)"() -> ("Value"=w41:u32)  [unwired: 2 in, 2 out]
    n160 = property on="DSP同时注入频点数" class="DigNum (严格)"() -> ("Value"=w31:u32)  [unwired: 2 in, 2 out]
    n161 = property on="响应(2号)端口类型" class="Ring (严格)"() -> ("Value"=w26:u8)  [unwired: 2 in, 2 out]
    n162 = property on="密度常数 dens" class="DigNum (严格)"() -> ("Value"=w40:dbl)  [unwired: 2 in, 2 out]
    n163 = Bundle("Value"=w43, "Value"=w42, "Value"=w41, "Value"=w40, "Value"=w39, "Value"=w25, "Value"=w27, "Value"=w26, "Value"=w28, "Value"=w29, "Value"=w30, "Value"=w31) -> (w37:T14)  [unwired: 1 in]
    n164 = Not Equal?(x=w38, y=w37) -> (x != y?=w35:T15)
    n165 = Cluster To Array(cluster=w35) -> (array=w36:bool[])
    n166 = Or Array Elements(Boolean array=w36) -> (logical OR=w34:bool)
    n167 = case shown="真" w34 {
      tunnel: w15 -> [w59 _]
      tunnel: w17 -> [w60 _]
      tunnel: [w60 w64] -> w32
      tunnel: [w62 w82] -> w23
      tunnel: [w61 w80] -> w24
      tunnel: w20 -> [w61 _]
      tunnel: w18 -> [w62 _]
      tunnel: w14 -> [w58 _]
      tunnel: [w59 w68] -> w22
      tunnel: [w58 w69] -> w21
      tunnel: [w57 w72] -> w19
      tunnel: w16 -> [w57 _]
      tunnel: w12 -> [w56 _]
      tunnel: [w56 w63] -> w13
      frame False {
      }
      frame True {
        # "当扫频设定改变时，更新设置"
        n168 = property on="注入(1号)端口类型" class="Ring (严格)"() -> ("Value"=w76:u8)  [unwired: 2 in, 2 out]
        n169 = property on="响应(2号)端口类型" class="Ring (严格)"() -> ("Value"=w75:u8)  [unwired: 2 in, 2 out]
        n170 = call "myFreqGen.vi"("f_dens"="密集中心频率 f_dens", "dens"="密度常数 dens", "f_min"="频率下限 f_min", "f_max"="频率上限 f_max", "N"="期望频点数 N0") -> ("freqs"=w79:i32[])  [unwired: 6 in]
        n171 = call "myFreqSymm.vi"("基频"="基波频率 f_fun", "注入(1号)端口类型"=w76, "Freqs in"=w79) -> ("Freqs out"=w78:i32[])  [unwired: 8 in]
        n172 = Array Size(array=w78) -> (size(s)=→"实际有效频点数 N":i32)
        n173 = call "myFreqSymp.vi"("基频"="基波频率 f_fun", "同步频率上限 f_tick_ref"="同步频率上限 f_tick_ref", "响应端口额外频率位移"="响应端口额外频率位移", "响应(2号)端口类型"=w75, "注入(1号)端口类型"=w76, "freqs in"=w78) -> ("f_mes_max"=w69:u32, "f_tick_min"=w68:u32, "freqs, measu, comps"=w64:i32[][])  [unwired: 3 in]
        n174 = call "myFreqGroup.vi"("基波频率"="基波频率 f_fun", "最大同时扫频数"="DSP同时注入频点数", "响应端口额外频率位移"="响应端口额外频率位移", "响应(2号)端口类型"=w75, "注入(1号)端口类型"=w76, "freqs_measu_coups"=w64) -> ("index group"=w63:i32[][], "freqs groups 3D"=w72:i32[][][])  [unwired: 4 in]
        n175 = call "myFreqPreview.vi"("f_tick_min"=w68, "同步频率上限 f_tick_ref"="同步频率上限 f_tick_ref", "f_mes_max"=w69, "测量周期数 n"="测量周期数 n", "freqs, measu, comps"=w64, "index group"=w63, "freqs groups"=w72) -> ("最大同时使用内存(kS)"=→"单频点最大使用内存":u64, "扫频点密度及其采样时长预览"=→"扫频点预览":T16, "group报告"=→"扫频点报告":string)  [unwired: 2 in]
        n176 = call "myOptionUI.vi"("响应(2号)端口类型"="响应(2号)端口类型", "注入(1号)端口类型"="注入(1号)端口类型", "同步相位来源"="同步相位来源", "测量模式"="测量模式") -> ("频点预览模式"=w83:u8, "if 需要设置触发"=w84:bool, "同步相位来源结果"=w82:u8, "if 显示同步相位选项"=w85:bool, "csv中存储列分别为"=→"csv中存储列分别为":string, "需要的示波器台数"=w80:u8, "测试选项说明"=→"测试选项说明":string, "if 显示端口类型选项"=w81:bool)
        n177 = property on="注入(1号)端口类型" class="Ring (严格)"("Visible"=w81) -> ()  [unwired: 2 in, 2 out]
        n178 = property on="响应(2号)端口类型" class="Ring (严格)"("Visible"=w81) -> ()  [unwired: 2 in, 2 out]
        n179 = property on="扫频点预览" class="XYGraph (严格)"("XScale.Mapping Mode"=w83, "YScale.Mapping Mode"=w83) -> ()  [unwired: 2 in, 2 out]
        n180 = property on="触发方向" class="Ring (严格)"("Visible"=w84) -> ()  [unwired: 2 in, 2 out]
        n181 = property on="触发阈值 (V)" class="DigNum (严格)"("Visible"=w84) -> ()  [unwired: 2 in, 2 out]
        n182 = property on="同步相位来源" class="Ring (严格)"("Visible"=w85) -> ()  [unwired: 2 in, 2 out]
      }
    }
    n183 = Wait (ms)(milliseconds to wait=u32 50) -> ()  [unwired: 1 out]
    n184 = Not(x="总电源") -> (.not. x?=w45:bool)
    n185 = case shown="真" "检验示波器" {
      tunnel: w24 -> [_ w49]
      frame False {
      }
      frame True {
        n186 = property on="注入(1号)端口类型" class="Ring (严格)"() -> ("Value"=w51:u8)  [unwired: 2 in, 2 out]
        n187 = property on="DSP同时注入频点数" class="DigNum (严格)"() -> ("Value"=w50:u32)  [unwired: 2 in, 2 out]
        n188 = property on="输出日志 log" class="Str"() -> ("Value"=w48:string)  [unwired: 2 in, 2 out]
        n189 = flat-sequence {
          tunnel: w47 -> [w54]
          frame #0 {
            n190 = local write "输出日志 log"(w54) -> ()
          }
          frame #1 {
            n191 = property on="输出日志 log" class="Str"("Text.Scroll Position"=inf) -> ()  [unwired: 2 in, 2 out]
          }
        }
        n192 = call "myPICO_CheckNum.vi"("需要的示波器台数"=w49, "当前log"=w48, "最大检测设备数"=i16 2, "最大同时扫频数"=w50, "注入(1号)端口类型"=w51) -> ("可以正常测量"=w52:bool, "更新log"=w47:string)  [unwired: 2 in, 3 out]
        n193 = property on="可以正常测量" class="Bool (严格)"("Value"=w52) -> ()  [unwired: 2 in, 2 out]
      }
    }
  }
  n194 = call "myFreqParamGen.vi"() -> ()  [unwired: 13 in, 3 out]
  "正在扫频" <- FALSE
  "输出日志 log" <- ""
